vi "RT_Network Read Loop.vi"(8 "error in":errorcluster, 11 "Main Data":T1) -> (0 "error out":errorcluster)   [LabVIEW 2018]
uses:
  Data Def/RT_Main Data.ctl
  Data Def/RT_FPGA VI Reference.ctl
  Data Def/RT_Request Data.ctl
  <vilib>/Platform/TimedLoop/XDataNode/timing_clust.ctl
  <vilib>/Platform/TimedLoop/XDataNode/nitl_modes.ctl
  <vilib>/Platform/TimedLoop/XDataNode/wakeup.ctl
  Com/WebSockets/Data Def/WebSocket Manerger Method.ctl
  <vilib>/platform/TimedLoop/XDataNode/XDataNode.xnode
  <vilib>/Platform/TimedLoop/XDataNode/XDNodeRunTimeDep.lvlib
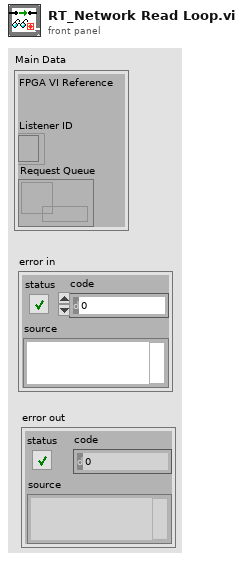
[diagram p1: front panel]
types:
  T1 = typedef "RT_Main Data.ctl" = cluster{"FPGA VI Reference":T2, "Listener ID":refnum<k5>, "Request Queue":refnum<queue>}
  T2 = typedef "RT_FPGA VI Reference.ctl" = refnum<k20>
  T3 = typedef "XDNodeRunTimeDep.lvlib/timing_clust.ctl" = cluster{"Expected End [f-1]":u64, "Actual End [f-1]":u64, "Finished Late? [f-1]":bool, "Expected End [i-1]":u64, "Actual End [i-1]":u64, "Finished Late? [i-1]":bool, "Expected Start [i]":u64, "Actual Start [i]":u64, "Expected Start [f]":u64, "Actual Start [f]":u64, "Source Name":string, "Structure Name":string, "Period":i64, "Deadline":i64, "Offset":i64, "Start":i64, "Priority":i32, "Timeout":i32, "Mode":T4, "Wakeup Reason":T5, "Error":errorcluster, "Source Type":string, "Secondary Source Type":string, "Global End Time":u64, "Global Start Time":u64, "Frame Duration":u64, "Iteration Duration":u64, "Assigned CPU":i32, "I/O Scan Engine Mode":u32}
  T4 = typedef "XDNodeRunTimeDep.lvlib/nitl_modes.ctl" = enum32{"No Change", "Process missed periods, maintain original phase", "Discard missed periods, maintain original phase", "Process missed periods, ignore original phase", "Discard missed periods, ignore original phase"}
  T5 = typedef "XDNodeRunTimeDep.lvlib/wakeup.ctl" = enum32{"Normal", "Aborted", "Asynchronous wakeup", "Timing source error", "Timed loop error", "Timeout"}
  T6 = typedef "WebSocket Manerger Method.ctl" = enum16{"Initialize", "Add Connection", "Get Connections", "Close Connection", "Close All"}
  T7 = typedef "RT_Request Data.ctl" = cluster{"Connection ID":refnum<k5>, "Command":string, "Data":string}
  T8 = typedef "Websocket Command.ctl" = cluster{"Command":string, "Data":string}
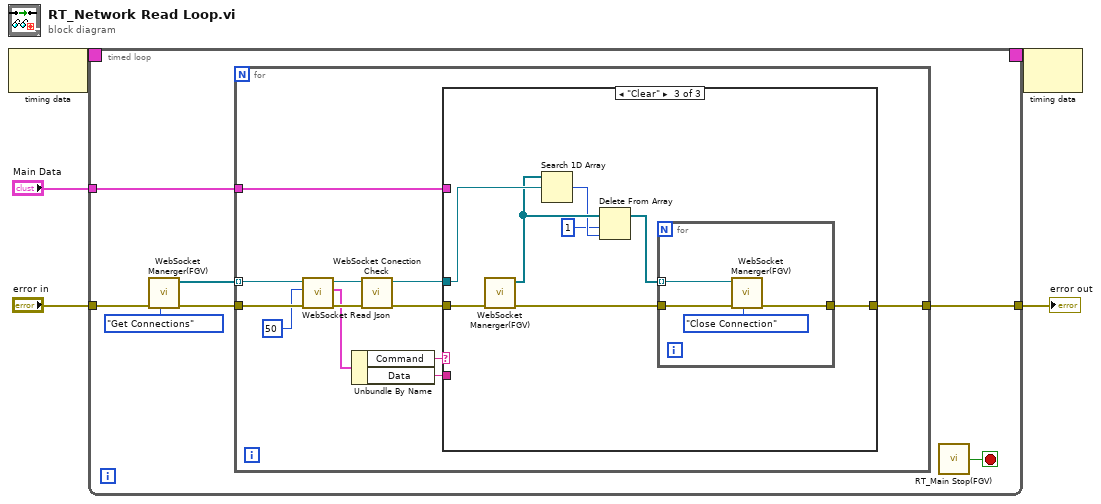
[diagram p0: block diagram]
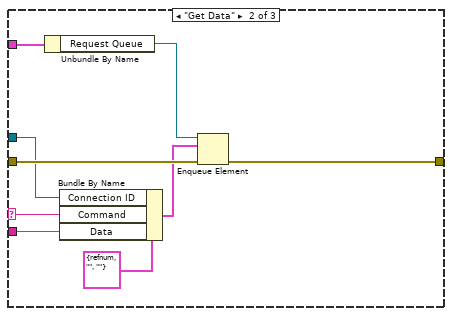
[diagram p3: hidden frame]
diagram:
  n1 = node-c288() -> (w4:T3)  [unwired: 1 in]
  n2 = timed-loop {
    tunnel: "error in" -> [w12]
    timing: w4 -> [_]
    timing-out: [_] -> w3
    tunnel: "Main Data" -> [w9]
    tunnel: [w8] -> w1
    stop <- w7 stop-if-true
    n3 = call "WebSocket Manerger(FGV).vi"("WebSocket Manerger Method"=WebSocket_Manerger_Method."Get Connections", "error in"=w12) -> ("error out"=w10:errorcluster, "connection Out"=w6:refnum<k5>[])  [unwired: 8 in]
    n4 = for {
      tunnel: w10 -> [w24]
      tunnel: w9 -> [w16]
      tunnel: [w14] -> w8
      tunnel: w6 -> [w13] mode=indexing
      n5 = call "WebSocket Read Json.vi"("error in"=w24, "timeout ms (5000)"=50, "WebSocket Connection in"=w13) -> ("error out"=w22:errorcluster, "Websocket Command"=w20:T8, "WebSocket Connection out"=w21:refnum<k5>)  [unwired: 6 in]
      n6 = Unbundle By Name(w20) -> ("Command"=w18:string, "Data"=w17:string)
      n7 = call "WebSocket Conection Check.vi"("error in"=w22, "Connection In"=w21) -> ("error out"=w19:errorcluster, "Connection Out"=w15:refnum<k5>)  [unwired: 8 in]
      n8 = case shown="\"Clear\"" w18 {
        selector: w18 -> [_ w30 _]
        tunnel: w19 -> [w25 w33 w42]
        tunnel: w17 -> [_ w29 _]
        tunnel: w16 -> [_ w34 _]
        tunnel: w15 -> [_ w28 w41]
        tunnel: [w25 w26 w35] -> w14
        frame Default {
        }
        frame "Get Data" {
          n9 = Unbundle By Name(w34) -> ("Request Queue"=w32:refnum<queue>)
          n10 = Bundle By Name(cluster=T7 {"Connection ID"=refnum, "Command"="", "Data"=""} ("element"), "Connection ID"=w28, "Command"=w30, "Data"=w29) -> (w27:T7)
          n11 = Enqueue Element(queue=w32, element=w27, error in (no error)=w33) -> (error out=w26:errorcluster)  [unwired: 1 in, 2 out]
        }
        frame "Clear" {
          n12 = call "WebSocket Manerger(FGV).vi"("error in"=w42) -> ("error out"=w37:errorcluster, "connection Out"=w40:refnum<k5>[])  [unwired: 9 in]
          n13 = Search 1D Array(1D array=w40, element=w41) -> (index of element=w39:i32)  [unwired: 1 in]
          n14 = Delete From Array(array=w40, length=1, index=w39) -> (array with subset deleted=w36:refnum<k5>[])  [unwired: 1 out]
          n15 = for {
            tunnel: w37 -> [w46]
            tunnel: w36 -> [w44] mode=indexing
            tunnel: [w43] -> w35
            n16 = call "WebSocket Manerger(FGV).vi"("WebSocket Manerger Method"=WebSocket_Manerger_Method."Close Connection", "error in"=w46, "connection In"=w44) -> ("error out"=w43:errorcluster)  [unwired: 7 in, 1 out]
          }
        }
      }
    }
    n17 = call "RT_Main Stop(FGV).vi"() -> ("Stop Out"=w7:bool)  [unwired: 4 in]
  }
  "error out" <- w1
  n18 = node-c288(w3) -> ()  [unwired: 1 out]
